vi "testing odor and manifold configuration_v3.vi"() -> ()   [LabVIEW 2021]
uses:
  type-defs/odor color (type def).ctl
  type-defs/odor selection (type def).ctl
  type-defs/odor info cluster (type def).ctl
  type-defs/odor description array (type def).ctl
  type-defs/port number (type def).ctl
  type-defs/single port single odor cluster.ctl
  type-defs/manifold selection.ctl
  type-defs/manifold configuration cluster (type def).ctl
  type-defs/manifold configuration cluster array (type def).ctl
panel:
  in  "load config":bool
  in  "save config":bool
  out "cycle number":i32
  in  "odor descriptions":T1
  in  "stimulator configuration":T5
  out "error out":errorcluster
  in  "error in (no error)":errorcluster
  in  "Stop":bool
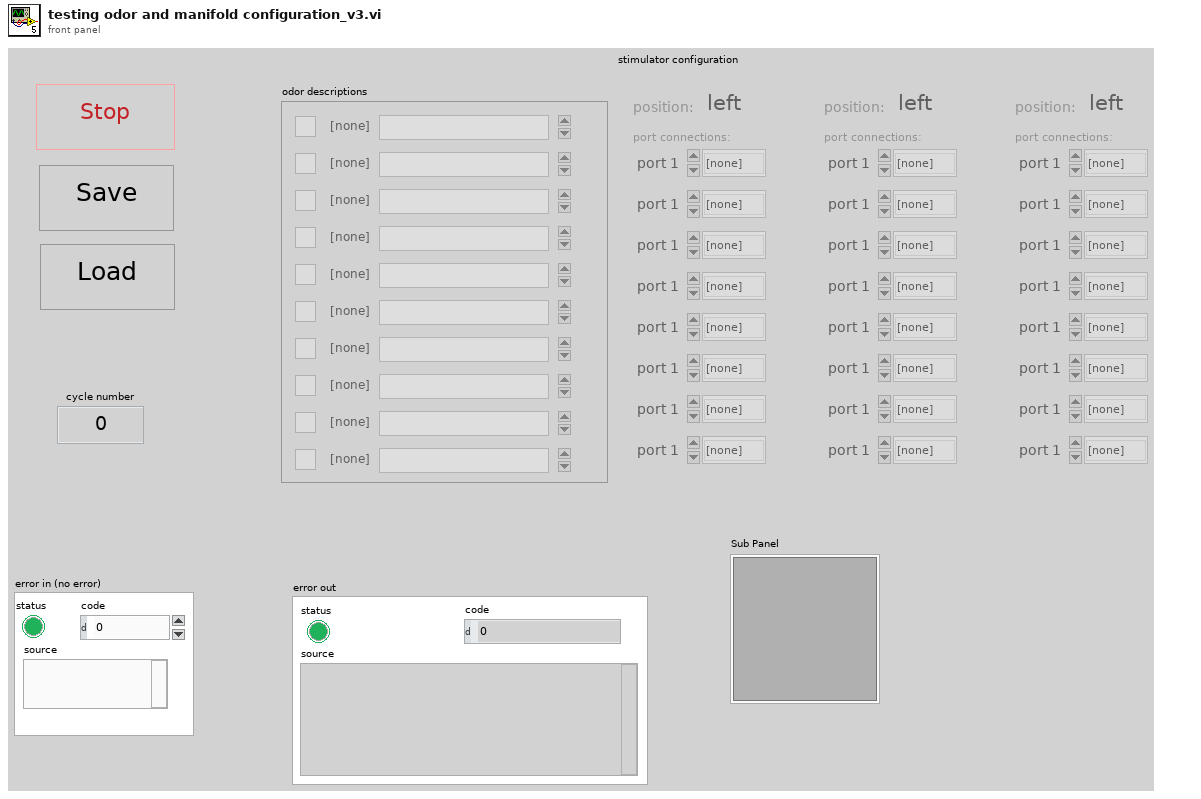
[diagram p1: front panel]
types:
  T1 = typedef "odor description array (type def).ctl" = T2[]
  T2 = typedef "odor info cluster (type def).ctl" = cluster{"odor channel":T3, "odor description":string, "odor color":T4, "odor channel active":bool}
  T3 = typedef "odor selection (type def).ctl" = enum16{"[none]", "odor 1", "odor 2", "odor 3", "odor 4", "odor 5", "odor 6", "odor 7", "odor 8", "odor 9", "odor 10"}
  T4 = typedef "odor color (type def).ctl" = u16
  T5 = typedef "manifold configuration cluster array (type def).ctl" = T6[]
  T6 = typedef "manifold configuration cluster (type def).ctl" = cluster{"position:":T7, "port connections:":T8[]}
  T7 = typedef "manifold selection.ctl" = enum16{"left", "middle", "right"}
  T8 = typedef "single port single odor cluster.ctl" = cluster{"port number":T9, "connected odor":T3, "error":bool, "odor color":T4}
  T9 = typedef "port number (type def).ctl" = enum16{"port 1", "port 2", "port 3", "port 4", "port 5", "port 6", "port 7", "port 8"}
  T10 = enum16{"big-endian, network order", "native, host order", "little-endian"}
  T11 = enum16{"open", "replace", "create", "open or create", "replace or create", "replace or create with confirmation"}
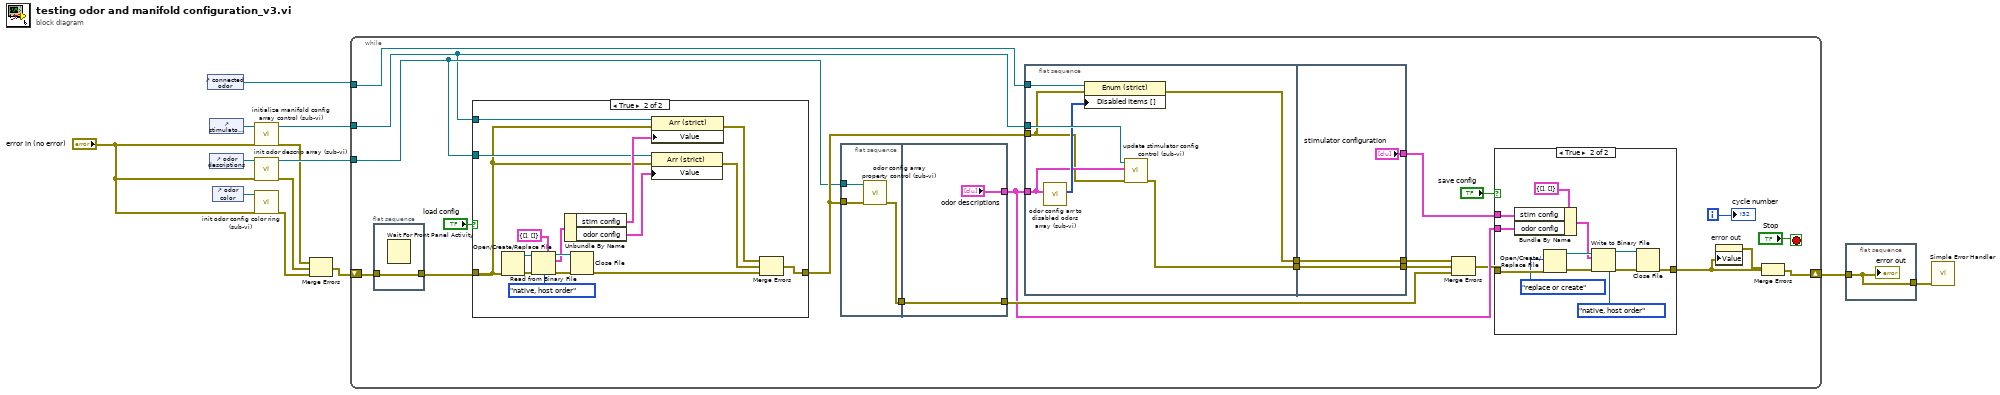
[diagram p0: block diagram]
diagram:
  n1 = control-ref of="connected odor"() -> (w4:refnum<vi>)
  n2 = control-ref of="stimulator configuration"() -> (w10:refnum<vi>)
  n3 = control-ref of="odor descriptions"() -> (w6:refnum<vi>)
  n4 = control-ref of="odor color"() -> (w5:refnum<vi>)
  n5 = call "initialize manifold config array control (sub-vi).vi"("error in (no error)"="error in (no error)", "stimulator config array refnum"=w10) -> ("error out"=w8:errorcluster, "stimulator config array refnum out"=w7:refnum<vi>)  [unwired: 8 in]
  n6 = call "init odor descrip array (sub-vi).vi"("error in (no error)"="error in (no error)", "array refnum"=w6) -> ("error out"=w11:errorcluster, "array refnum out"=w12:refnum<vi>)  [unwired: 8 in]
  n7 = call "init odor config color ring (sub-vi).vi"("error in (no error)"="error in (no error)", "ring refnum"=w5) -> ("error out"=w13:errorcluster)  [unwired: 8 in, 1 out]
  n8 = Merge Errors(w8, w11, w13) -> (w1:errorcluster)
  n9 = while {
    shift-right: [w33] -> w3
    shift-left: w1 -> [w27]
    tunnel: w7 -> [w14]
    tunnel: w12 -> [w15]
    tunnel: w4 -> [w19]
    i -> [w28]
    stop <- "Stop" stop-if-true
    n10 = flat-sequence {
      tunnel: w27 -> [w76]
      tunnel: [w76] -> w17
      frame #0 {
        n11 = Wait For Front Panel Activity() -> ()  [unwired: 3 in, 1 out]
      }
    }
    n12 = case shown="True" "load config" {
      tunnel: w17 -> [w36 w42]
      tunnel: [w36 w41] -> w18
      tunnel: w15 -> [_ w43]
      tunnel: w14 -> [_ w45]
      frame False {
      }
      frame True {
        n13 = Open/Create/Replace File(error in=w42) -> (refnum out=w51:refnum<file>, error out=w52:errorcluster)  [unwired: 5 in, 1 out]
        n14 = Read from Binary File(5:cluster{"stim config":T5, "odor config":T1} {"stim config"=[], "odor config"=[]} ("Cluster"), 8:w52, 9:T10."native, host order" ("byte order (0:big-endian, network order)"), 11:w51) -> (0:w50:errorcluster, 2:w46:cluster{"stim config":T5, "odor config":T1}, 3:w48:refnum<file>)  [unwired: 2 in, 1 out]
        n15 = Unbundle By Name(w46) -> ("stim config"=w44:T5, "odor config"=w38:T1)
        n16 = Close File(refnum=w48, error in=w50) -> (error out=w49:errorcluster)  [unwired: 1 out]
        n17 = property class="Arr (strict)"(reference=w43, error in=w42, "Value"=w38) -> (error out=w39:errorcluster)  [unwired: 1 out]
        n18 = property class="Arr (strict)"(reference=w45, error in=w42, "Value"=w44) -> (error out=w40:errorcluster)  [unwired: 1 out]
        n19 = Merge Errors(w40, w39, w49) -> (w41:errorcluster)
      }
    }
    n20 = flat-sequence {
      tunnel: w15 -> [w79]
      tunnel: w18 -> [w78]
      tunnel: [w77] -> w32
      tunnel: w32 -> [w81]
      tunnel: [w81] -> w31
      tunnel: ["odor descriptions"] -> w23
      frame #0 {
        n21 = call "odor config array property control (sub-vi).vi"("error in (no error)"=w78, "odor config array refnum"=w79) -> ("error out"=w77:errorcluster)  [unwired: 8 in, 1 out]
      }
      frame #1 {
      }
    }
    n22 = flat-sequence {
      tunnel: w19 -> [w72]
      tunnel: w14 -> [w71]
      tunnel: w23 -> [w68]
      tunnel: w18 -> [w66]
      tunnel: [w69] -> w26
      tunnel: [w67] -> w25
      tunnel: [w74] -> w29
      tunnel: [w75] -> w30
      tunnel: w26 -> [w75]
      tunnel: w25 -> [w74]
      tunnel: ["stimulator configuration"] -> w24
      frame #0 {
        n23 = call "odor config arr to disabled odors array (sub-vi).vi"("odor descriptions"=w68) -> ("Disabled Items []"=w70:i32[])  [unwired: 10 in]
        n24 = property class="Enum (strict)"(reference=w72, error in=w66, "Disabled Items []"=w70) -> (error out=w69:errorcluster)  [unwired: 1 out]
        n25 = call "update stimulator config control (sub-vi).vi"("error in (no error)"=w66, "re/initialize (F)"=w68, "manifold config array refnum"=w71) -> ("error out"=w67:errorcluster)  [unwired: 6 in, 2 out]
      }
      frame #1 {
      }
    }
    n26 = Merge Errors(w30, w29, w31) -> (w22:errorcluster)
    n27 = case shown="True" "save config" {
      tunnel: w24 -> [_ w65]
      tunnel: w23 -> [_ w64]
      tunnel: w22 -> [w53 w62]
      tunnel: [w53 w57] -> w21
      frame False {
      }
      frame True {
        n28 = Bundle By Name(cluster=cluster{"stim config":T5, "odor config":T1} {"stim config"=[], "odor config"=[]} ("Cluster"), "stim config"=w65, "odor config"=w64) -> (w59:cluster{"stim config":T5, "odor config":T1})
        n29 = Open/Create/Replace File(error in=w62, operation (0:open)=T11."replace or create") -> (refnum out=w60:refnum<file>, error out=w61:errorcluster)  [unwired: 4 in, 1 out]
        n30 = Write to Binary File(file (use dialog)=w60, data=w59, error in=w61, 9:T10."native, host order" ("byte order (0:big-endian, network order)")) -> (refnum out=w56:refnum<file>, error out=w58:errorcluster)  [unwired: 2 in, 1 out]
        n31 = Close File(refnum=w56, error in=w58) -> (error out=w57:errorcluster)  [unwired: 1 out]
      }
    }
    n32 = property on="error out" class="Clust (strict)"("Value"=w21) -> (error out=w34:errorcluster)  [unwired: 2 in, 1 out]
    n33 = Merge Errors(w34, w21) -> (w33:errorcluster)
    "cycle number" <- w28
  }
  n34 = flat-sequence {
    tunnel: w3 -> [w82]
    tunnel: [w82] -> w2
    frame #0 {
      "error out" <- w82
    }
  }
  n35 = call <vilib>:"Simple Error Handler.vi"("error in (no error)"=w2) -> ()  [unwired: 4 in, 5 out]
